vi "refnum variable.vi"(7 "action":T1, 8 "error in (no error)":errorcluster, 10 "reference in":refnum<k24>) -> (0 "error out":errorcluster, 2 "reference in 2":refnum<k24>)   [LabVIEW 2018]
uses:
  C:/Project/SerialSectionOCT/SerialSectOCT/Labview Software/Thorlabs.MotionControl.Controls.dll
  Thorlabs.MotionControl.Controls.dll
  refnum control.ctl
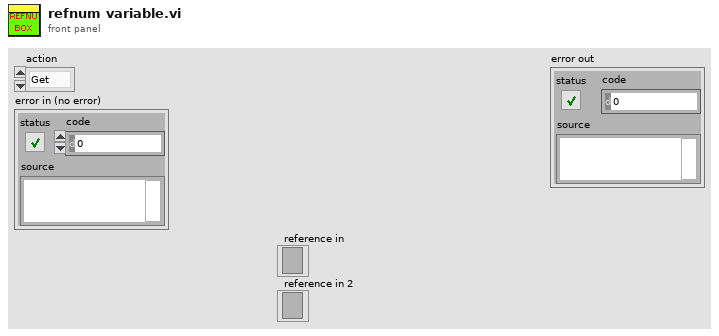
[diagram p1: front panel]
types:
  T1 = typedef "refnum control.ctl" = enum16{"Get", "Init"}
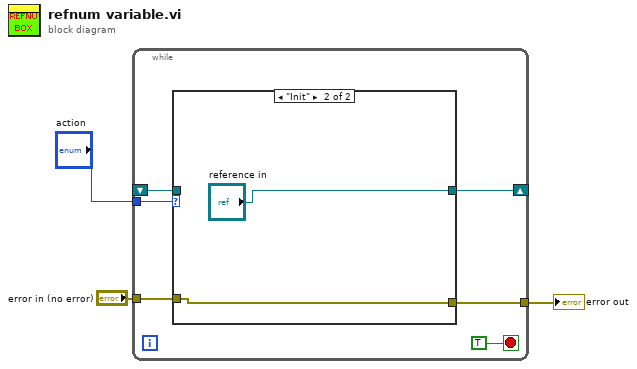
[diagram p0: block diagram]
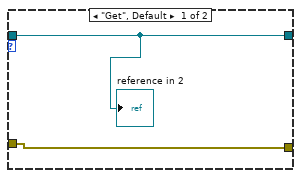
[diagram p2: hidden frame]
diagram:
  n1 = while {
    tunnel: "action" -> [w9]
    shift-right: [w8] -> _
    shift-left: _ -> [w7]
    tunnel: "error in (no error)" -> [w5]
    tunnel: [w4] -> w1
    stop <- TRUE stop-if-true
    n2 = case shown="\"Init\"" w9 {
      tunnel: [w11 "reference in"] -> w8
      tunnel: w7 -> [w11 _]
      tunnel: w5 -> [w10 w12]
      tunnel: [w10 w12] -> w4
      frame "Get", Default {
        "reference in 2" <- w11
      }
      frame "Init" {
      }
    }
  }
  "error out" <- w1
